vi "Run Next Step.vi"(8 "error in (no error)":errorcluster, 11 "SequencingModel in":refnum<class "SequencingModel.lvclass">) -> (0 "error out":errorcluster, 3 "SequencingModel out":refnum<class "SequencingModel.lvclass">)   [LabVIEW 2017, in "SequencingModel.lvlib" / "SequencingModel.lvclass"]
uses:
  <vilib>/gpm_packages/@cs/example/Dynamic Viewables/SequencingModel/SequencingModel.lvclass
  C:/Program Files/National Instruments/LabVIEW 2017/vi.lib/gpm_packages/@cs/mva-core/Source/IModel/IModel/IModel.lvclass
  <vilib>/gpm_packages/@cs/example/Dynamic Viewables/SequencingModel/SequencingModel.lvclass/SequencingModel.ctl
  <vilib>/gpm_packages/@cs/mva-core/Source/IObserver/IObserver/IObserver.lvclass/IObserver.ctl
  <vilib>/gpm_packages/@cs/mva-core/Source/IModel/IModel/IModel.lvclass/IModel.ctl
  <vilib>/gpm_packages/@cs/mva-core/Source/IMediator/PublishRequest/PublishRequest.lvclass/PublishRequest.ctl
  <vilib>/gpm_packages/@cs/mva-core/Source/IMediator/IMediator Messages/Publish Msg/Publish Msg.lvclass/Publish Msg.ctl
  <vilib>/gpm_packages/@cs/actor-framework-messages/Source/RoundTripMessage/RoundTripMessage.lvclass/RoundTripMessage.ctl
  <vilib>/ActorFramework/Message Enqueuer/Message Enqueuer.lvclass/Message Enqueuer.ctl
  <vilib>/gpm_packages/@cs/mva-core/Source/IMediator/IMediator Messages/Publish Msg/Send Pre-Addressed Publish.vi
  <vilib>/gpm_packages/@cs/mva-core/Source/IObserver/IObserver/Read Unique ID.vi
  <vilib>/gpm_packages/@cs/mva-core/Source/IMediator/PublishRequest/Pack Publish Request.vi
  <vilib>/gpm_packages/@cs/actor-framework-messages/Source/RoundTripMessage/Return Round-Trip Message.vi
  <vilib>/ActorFramework/Message Enqueuer/Enqueue.vi
  <vilib>/gpm_packages/@cs/mva-core/Source/IModel/IModel/IModel.lvclass
  C:/Program Files/National Instruments/LabVIEW 2017/vi.lib/ActorFramework/Actor/Actor.lvclass
  C:/Program Files/National Instruments/LabVIEW 2017/vi.lib/gpm_packages/@cs/mva-core/Source/IObserver/IObserver/IObserver.lvclass
  <vilib>/gpm_packages/@cs/mva-core/Source/IMediator/IMediator Messages/Publish Msg/Publish Msg.lvclass
  C:/Program Files/National Instruments/LabVIEW 2017/vi.lib/gpm_packages/@cs/actor-framework-messages/Source/RoundTripMessage/RoundTripMessage.lvclass
  <vilib>/gpm_packages/@cs/actor-framework-messages/Source/RoundTripMessage/RoundTripMessage.lvclass
  C:/Program Files/National Instruments/LabVIEW 2017/vi.lib/ActorFramework/Message/Message.lvclass
  <vilib>/Utility/error.llb/Error Cluster From Error Code.vi
  <vilib>/ActorFramework/Message Priority Queue/Priority Enqueue.vi
  <vilib>/gpm_packages/@cs/mva-core/Source/IMediator/PublishRequest/PublishRequest.lvclass
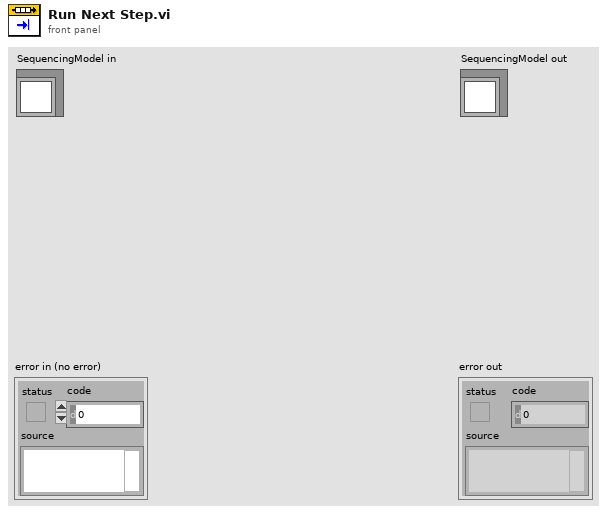
[diagram p1: front panel]
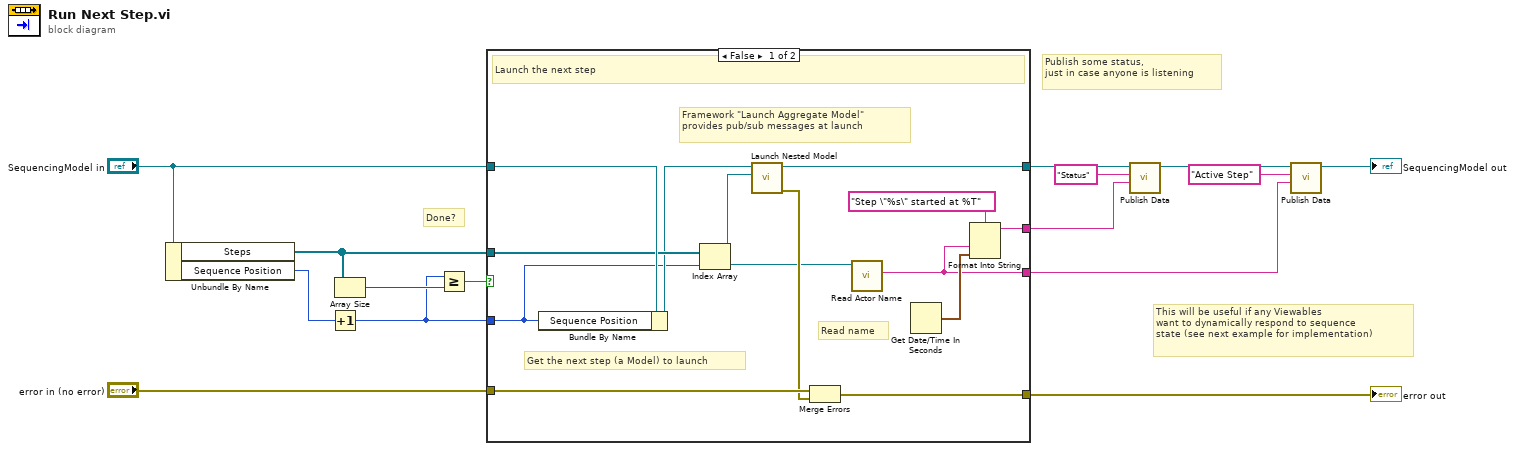
[diagram p0: block diagram]
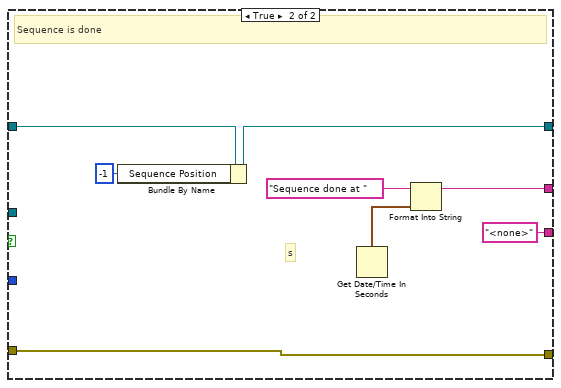
[diagram p2: hidden frame]
diagram:
  # "This will be useful if any Viewables\nwant to dynamically respond to sequence\nstate (see next example for implementation)"
  # "Done?"
  # "Publish some status,\njust in case anyone is listening"
  n1 = Unbundle By Name("SequencingModel in") -> ("Steps"=w9:refnum<class "IModel.lvclass">[], "Sequence Position"=w7:i32)
  n2 = Increment(x=w7) -> (x+1=w5:i32)
  n3 = Array Size(array=w9) -> (size(s)=w8:i32)
  n4 = Greater Or Equal?(x=w5, y=w8) -> (x >= y?=w6:bool)
  n5 = case shown="False" w6 {
    tunnel: "error in (no error)" -> [w28 w32]
    tunnel: "SequencingModel in" -> [w27 w36]
    tunnel: [w18 w31] -> w13
    tunnel: [w26 w32] -> w12
    tunnel: [w23 w33] -> w10
    tunnel: w9 -> [w22 _]
    tunnel: w5 -> [w20 _]
    tunnel: [w16 "<none>" ("Name")] -> w1
    frame False {
      # "Read name"
      # "Framework \"Launch Aggregate Model\"\nprovides pub/sub messages at launch"
      # "Get the next step (a Model) to launch"
      # "Launch the next step"
      n6 = Bundle By Name(cluster=w27, "Sequence Position"=w20) -> (w21:refnum<class "SequencingModel.lvclass">)
      n7 = Index Array(array=w22, index=w20) -> (element=w17:refnum<class "IModel.lvclass">)
      n8 = call-dynamic "Launch Nested Model.vi"("Model to Launch"=w17, "IModel in"=w21) -> ("error out"=w25:errorcluster, "IModel out"=w18:refnum<class "SequencingModel.lvclass">)  [unwired: 7 in, 1 out]
      n9 = Merge Errors(w28, w25) -> (w26:errorcluster)
      n10 = call <vilib>:"Read Actor Name.vi"("Actor in"=w17) -> ("Name"=w16:string)  [unwired: 10 in]
      n11 = Get Date/Time In Seconds() -> (seconds since 1Jan1904=w24:timestamp)
      n12 = Format Into String(format string="Step \"%s\" started at %T", w16, w24) -> (resulting string=w23:string)  [unwired: 2 in, 1 out]
    }
    frame True {
      # "s"
      # "Sequence is done"
      n13 = Bundle By Name(cluster=w36, "Sequence Position"=-1) -> (w31:refnum<class "SequencingModel.lvclass">)
      n14 = Get Date/Time In Seconds() -> (seconds since 1Jan1904=w34:timestamp)
      n15 = Format Into String(initial string="Sequence done at ", w34) -> (resulting string=w33:string)  [unwired: 2 in, 1 out]
    }
  }
  "error out" <- w12
  n16 = call <vilib>:"Publish Data.vi"("Data to Publish"=w10, "Datum Name"="Status", "IModel in"=w13) -> ("IModel out"=w3:refnum<class "SequencingModel.lvclass">)  [unwired: 7 in, 1 out]
  n17 = call <vilib>:"Publish Data.vi"("Data to Publish"=w1, "Datum Name"="Active Step", "IModel in"=w3) -> ("IModel out"=→"SequencingModel out":refnum<class "SequencingModel.lvclass">)  [unwired: 7 in, 1 out]
